vi "MB Update Registers.vi"(8 "error in (no error)":errorcluster, 11 "Modbus Data Unit In":T1={"Function Code"=1, "Data"=[]} {"Function Code" items=["Read Coils"=1, "Read Discrete Inputs"=2, "Read Holding Registers"=3, "Read Input Registers"=4, "Write Single Coil"=5, "Write Single Register"=6, "Read Exception Status"=7, "Write Multiple Coils"=15, "Write Multiple Registers"=16]; "Data" format="%.0x"}) -> (0 "error out":errorcluster, 3 "Modbus Data Unit Out":T1={"Function Code"=1, "Data"=[]} {"Function Code" items=["Read Coils"=1, "Read Discrete Inputs"=2, "Read Holding Registers"=3, "Read Input Registers"=4, "Write Single Coil"=5, "Write Single Register"=6, "Read Exception Status"=7, "Write Multiple Coils"=15, "Write Multiple Registers"=16]; "Data" format="%.0x"})   [LabVIEW 2023, in "Voegtlin_NI_SMART_Modbus_Drivers.lvlib"]
uses:
  Voegtlin_NI_SMART_Modbus_Drivers.lvlib
  MB Modbus Data Unit.ctl
  MB Globals.vi
panel:
  # "VI Name: MB Serial Master Transceive.vi\nPurpose: Performs a MODBUS query and format\nMODBUS Data Unit for the answer.\nReentrant."
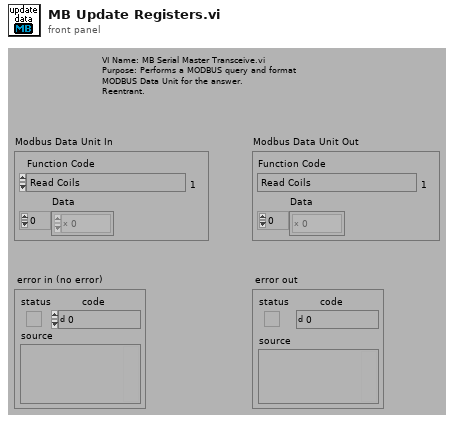
[diagram p1: front panel]
types:
  T1 = typedef "Voegtlin_NI_SMART_Modbus_Drivers.lvlib/MB Modbus Data Unit.ctl" = cluster{"Function Code":u8, "Data":u8[]}
  T2 = enum16{"Discrete Inputs", "Coils", "Input Registers", "Holding Registers"}
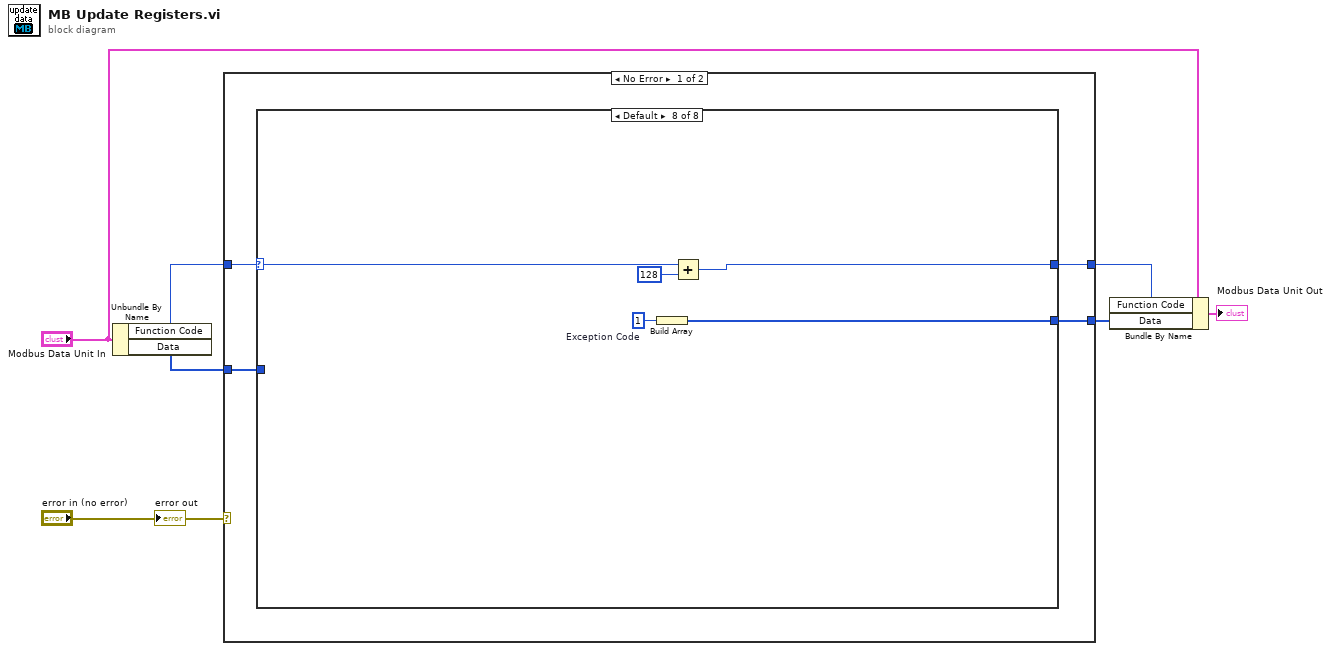
[diagram p0: block diagram]
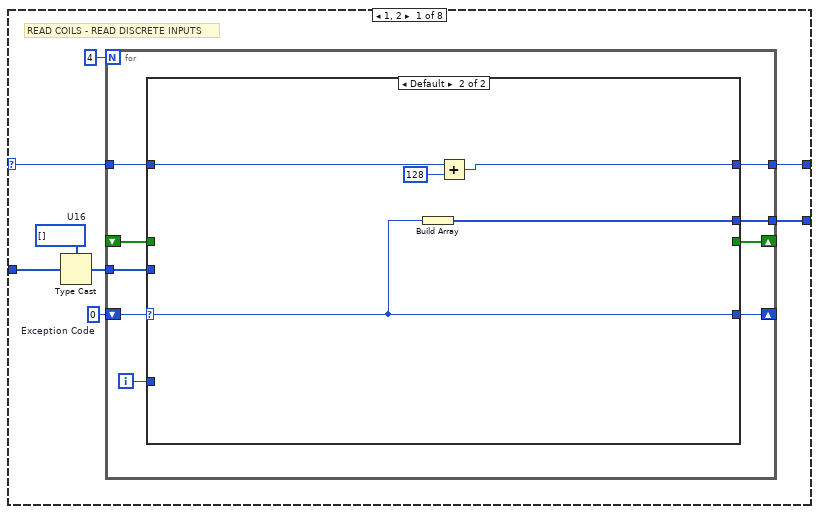
[diagram p2: hidden frame]
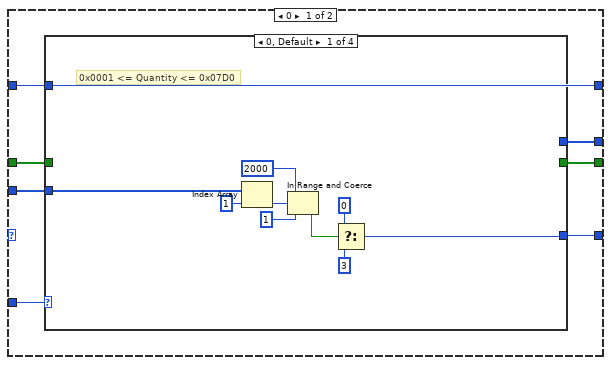
[diagram p3: hidden frame]
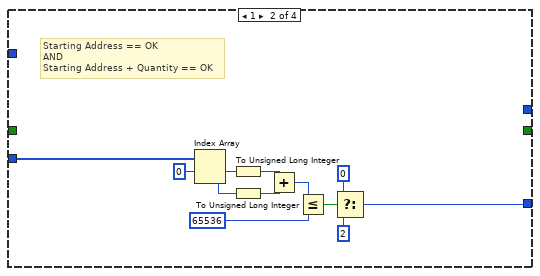
[diagram p4: hidden frame]
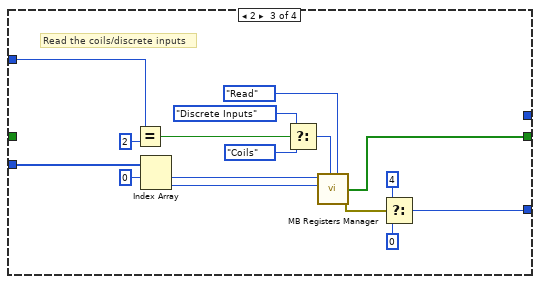
[diagram p5: hidden frame]
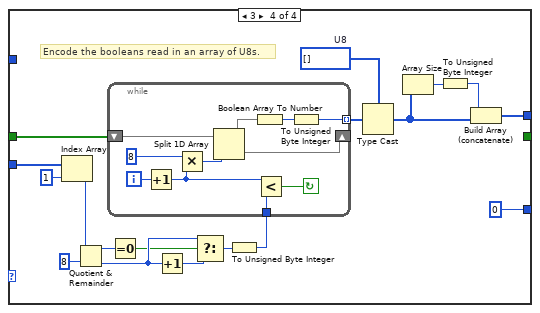
[diagram p6: hidden frame]
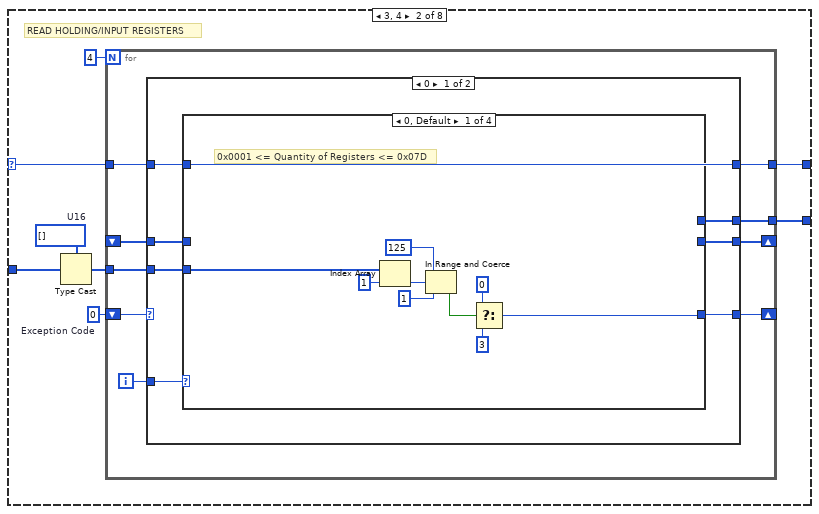
[diagram p7: hidden frame]
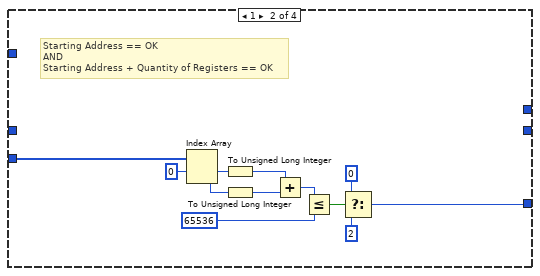
[diagram p8: hidden frame]
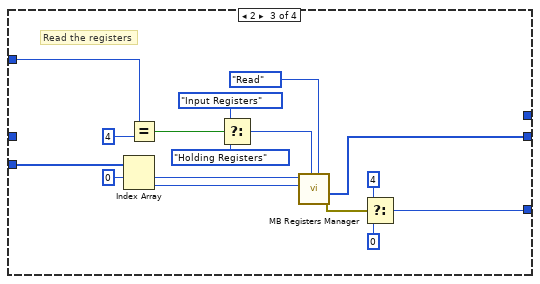
[diagram p9: hidden frame]
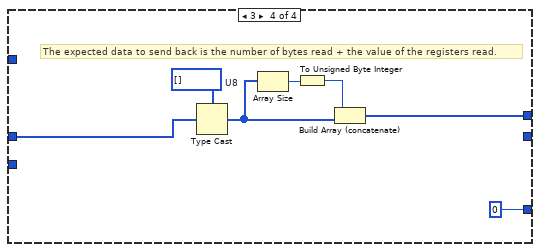
[diagram p10: hidden frame]
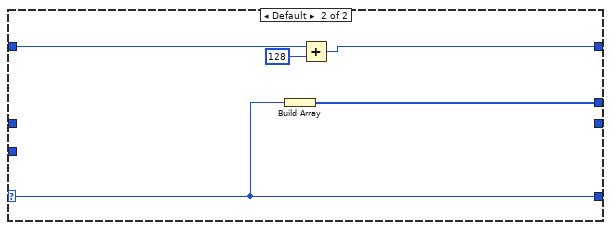
[diagram p11: hidden frame]
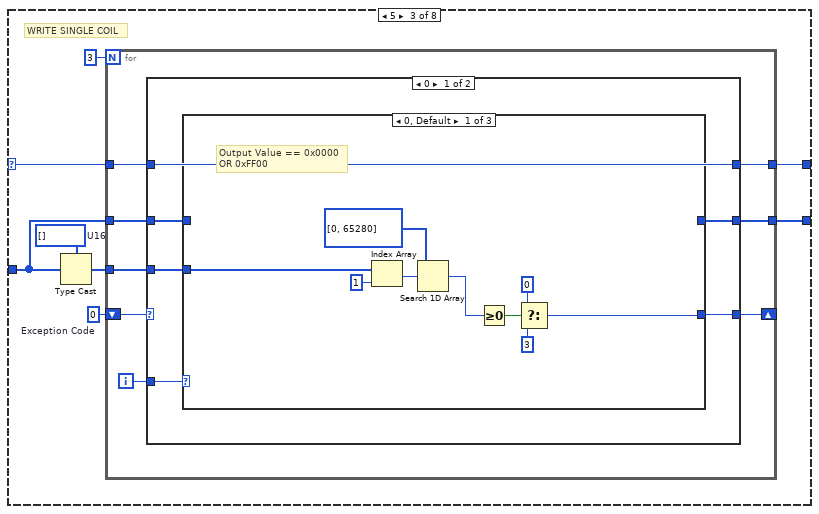
[diagram p12: hidden frame]
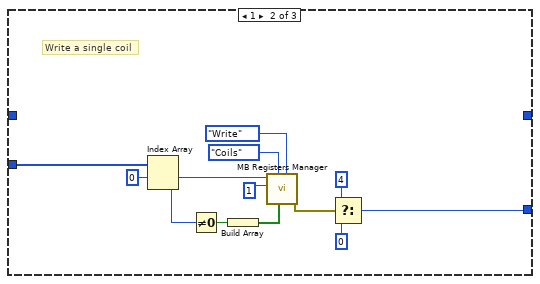
[diagram p13: hidden frame]
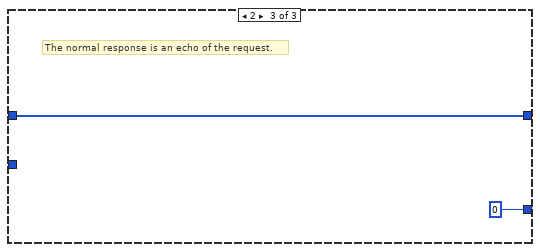
[diagram p14: hidden frame]
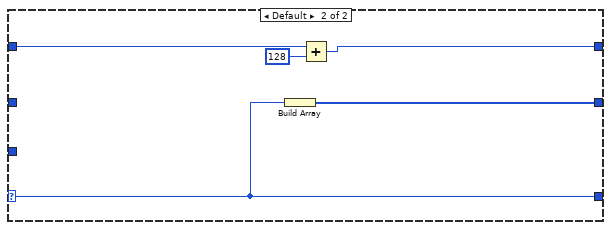
[diagram p15: hidden frame]
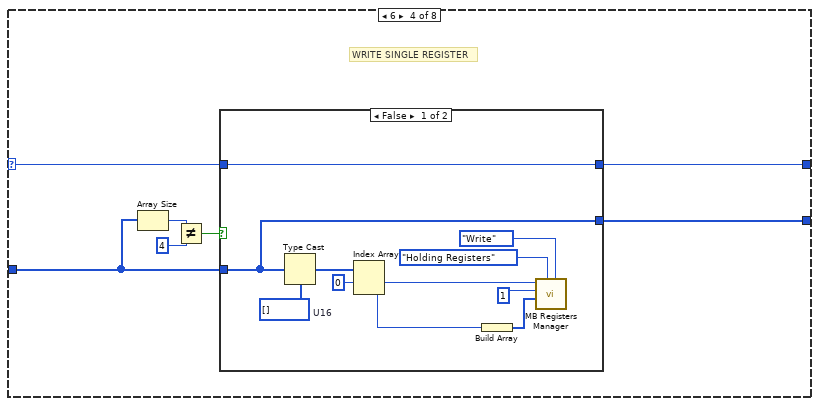
[diagram p16: hidden frame]
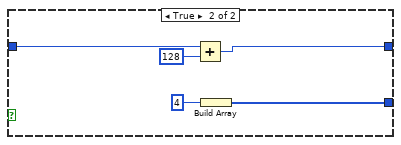
[diagram p17: hidden frame]
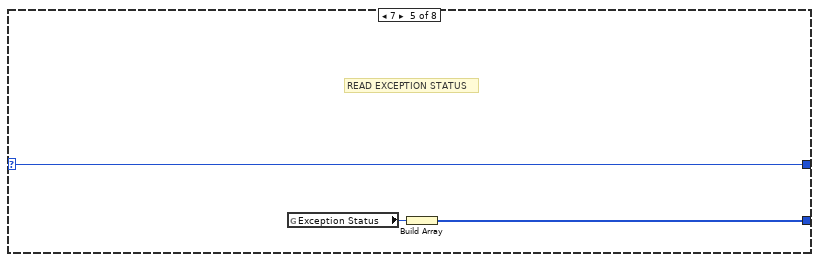
[diagram p18: hidden frame]
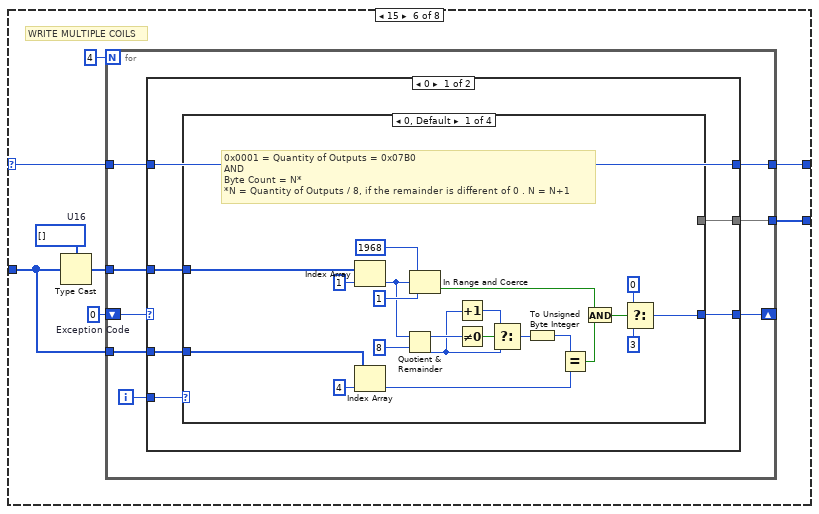
[diagram p19: hidden frame]
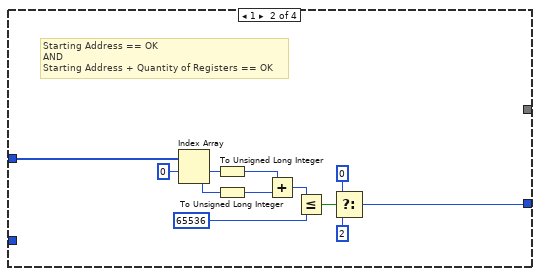
[diagram p20: hidden frame]
diagram:
  n1 = Unbundle By Name("Modbus Data Unit In") -> ("Function Code"=w3:u8, "Data"=w7:u8[])
  n2 = case shown="No Error" "error in (no error)" {
    tunnel: [w11 w421] -> w5
    tunnel: w7 -> [w10 w421]
    tunnel: w3 -> [w9 w420]
    tunnel: [w8 w420] -> w2
    frame No Error {
      n3 = case shown="Default" w9 {
        selector: w9 -> [w12 w107 w181 w237 w255 w258 w342 w418]
        tunnel: w10 -> [w16 w111 w180 w234 _ w257 w341 _]
        tunnel: [w15 w110 w184 w235 w256 w261 w345 w416] -> w11
        tunnel: [w13 w108 w182 w236 w255 w259 w343 w417] -> w8
        frame 1, 2 {
          w18 = u16[] []  # U16
          w19 = u8 0  # Exception Code
          # "READ COILS - READ DISCRETE INPUTS"
          n4 = Type Cast(type=w18, x=w16) -> (*(type *) &x=w17:u16[])
          n5 = for {
            N: 4 -> [_]
            shift-right: [w26] -> _
            shift-left: w19 -> [w28]
            tunnel: w17 -> [w27]
            shift-right: [w25] -> _
            shift-left: _ -> [w24]
            tunnel: [w23] -> w15
            tunnel: [w21] -> w13
            tunnel: w12 -> [w20]
            i -> [w22]
            n6 = case shown="Default" w28 {
              selector: w28 -> [_ w106]
              tunnel: w27 -> [w35 _]
              tunnel: [w34 w106] -> w26
              tunnel: [w33 _] -> w25
              tunnel: w24 -> [w32 _]
              tunnel: [w31 w105] -> w23
              tunnel: w22 -> [w30 _]
              tunnel: [w29 w102] -> w21
              tunnel: w20 -> [w29 w104]
              frame 0 {
                n7 = case shown="0, Default" w30 {
                  tunnel: w35 -> [w43 w55 w71 w89]
                  tunnel: [w38 w54 w63 u8 0] -> w34
                  tunnel: [_ _ w67 _] -> w33
                  tunnel: w32 -> [_ _ _ w75]
                  tunnel: [_ _ _ w74] -> w31
                  tunnel: w29 -> [_ _ w62 _]
                  frame 0, Default {
                    # "0x0001 <= Quantity <= 0x07D0"
                    n8 = Index Array(array=w43, index=1) -> (element=w42:u16)
                    n9 = In Range and Coerce(upper limit=u16 2000, x=w42, lower limit=u16 1) -> (In Range?=w39:bool)  [unwired: 1 out]
                    n10 = Select(t=u8 0, s=w39, f=u8 3) -> (s? t:f=w38:u8)
                  }
                  frame 1 {
                    # "Starting Address == OK\nAND\nStarting Address + Quantity == OK"
                    n11 = Index Array(array=w55, index #1=0 ("index")) -> (element #1=w51:u16, element #2=w48:u16)  [unwired: 1 in]
                    n12 = To Unsigned Long Integer(number=w51) -> (unsigned 32bit integer=w46:u32)
                    n13 = To Unsigned Long Integer(number=w48) -> (unsigned 32bit integer=w47:u32)
                    n14 = Add(x=w46, y=w47) -> (x+y=w50:u32)
                    n15 = Less Or Equal?(x=w50, y=u32 65536 ("upper limit")) -> (x <= y?=w45:bool)
                    n16 = Select(t=u8 0, s=w45, f=u8 2) -> (s? t:f=w54:u8)
                  }
                  frame 2 {
                    # "Read the coils/discrete inputs"
                    n17 = Equal?(x=w62, y=u8 2) -> (x = y?=w60:bool)
                    n18 = Index Array(array=w71, index #1=0 ("index")) -> (element #1=w69:u16, element #2=w68:u16)  [unwired: 1 in]
                    n19 = Select(t=T2."Discrete Inputs" ("Table"), s=w60, f=T2."Coils" ("Table")) -> (s? t:f=w57:T2)
                    n20 = call "MB Registers Manager.vi"("Function"=enum16{"Init", "Read", "Write", "Read All"}."Read", "Table"=w57, "Length"=w68, "Start Address"=w69) -> ("error out"=w66:errorcluster, "Bits out"=w67:bool[])  [unwired: 3 in, 3 out]
                    n21 = Select(t=u8 4, s=w66, f=u8 0) -> (s? t:f=w63:u8)
                  }
                  frame 3 {
                    w77 = u8[] []  # U8
                    # "Encode the booleans read in an array of U8s."
                    n22 = Index Array(array=w89, index=1) -> (element=w82:u16)
                    n23 = Quotient & Remainder(x=w82, y=u16 8) -> (x-y*floor(x/y)=w84:u16, floor(x/y)=w87:u16)
                    n24 = Equal To 0?(x=w84) -> (x = 0?=w85:bool)
                    n25 = Increment(x=w87) -> (x+1=w86:u16)
                    n26 = Select(t=w87, s=w85, f=w86) -> (s? t:f=w88:u16)
                    n27 = To Unsigned Byte Integer(number=w88) -> (unsigned 8bit integer=w76:u8)
                    n28 = while {
                      shift-left: w75 -> [w92]
                      shift-right: [w93] -> _
                      tunnel: [w100] -> w81 mode=indexing
                      tunnel: w76 -> [w91]
                      i -> [w97]
                      stop <- w99 continue-if-true
                      n29 = Increment(x=w97) -> (x+1=w96:i32)
                      n30 = Multiply(x=8, y=w96) -> (x*y=w94:i32)
                      n31 = Split 1D Array(array=w92, index=w94) -> (first subarray=w98:bool[], second subarray=w93:bool[])
                      n32 = Boolean Array To Number(Boolean array=w98) -> (number=w101:u32)
                      n33 = Less?(x=w96, y=w91) -> (x < y?=w99:bool)
                      n34 = To Unsigned Byte Integer(number=w101) -> (unsigned 8bit integer=w100:u8)
                    }
                    n35 = Type Cast(type=w77, x=w81) -> (*(type *) &x=w79:u8[])
                    n36 = Array Size(array=w79) -> (size(s)=w80:i32)
                    n37 = To Unsigned Byte Integer(number=w80) -> (unsigned 8bit integer=w78:u8)
                    n38 = Build Array (concatenate)(w78, w79) -> (w74:u8[])
                  }
                }
              }
              frame Default {
                n39 = Build Array(w106) -> (w105:u8[])
                n40 = Add(x=w104, y=u8 128) -> (x+y=w102:u8)
              }
            }
          }
        }
        frame 3, 4 {
          w113 = u16[] []  # U16
          w114 = u8 0  # Exception Code
          # "READ HOLDING/INPUT REGISTERS"
          n41 = Type Cast(type=w113, x=w111) -> (*(type *) &x=w112:u16[])
          n42 = for {
            N: 4 -> [_]
            shift-right: [w121] -> _
            shift-left: w114 -> [w123]
            tunnel: w112 -> [w122]
            shift-right: [w120] -> _
            shift-left: _ -> [w119]
            tunnel: [w118] -> w110
            tunnel: [w116] -> w108
            tunnel: w107 -> [w115]
            i -> [w117]
            n43 = case shown="0" w123 {
              selector: w123 -> [_ w179]
              tunnel: w122 -> [w130 _]
              tunnel: [w129 w179] -> w121
              tunnel: [w128 _] -> w120
              tunnel: w119 -> [w127 _]
              tunnel: [w126 w178] -> w118
              tunnel: w117 -> [w125 _]
              tunnel: [w124 w175] -> w116
              tunnel: w115 -> [w124 w177]
              frame 0 {
                n44 = case shown="0, Default" w125 {
                  tunnel: w130 -> [w138 w150 w166 _]
                  tunnel: [w133 w149 w159 u8 0] -> w129
                  tunnel: [_ _ w158 _] -> w128
                  tunnel: w127 -> [_ _ _ w168]
                  tunnel: [_ _ _ w169] -> w126
                  tunnel: w124 -> [_ _ w157 _]
                  frame 0, Default {
                    # "0x0001 <= Quantity of Registers <= 0x07D"
                    n45 = Index Array(array=w138, index=1) -> (element=w137:u16)
                    n46 = In Range and Coerce(upper limit=u16 125, x=w137, lower limit=u16 1) -> (In Range?=w134:bool)  [unwired: 1 out]
                    n47 = Select(t=u8 0, s=w134, f=u8 3) -> (s? t:f=w133:u8)
                  }
                  frame 1 {
                    # "Starting Address == OK\nAND\nStarting Address + Quantity of Registers == OK"
                    n48 = Index Array(array=w150, index #1=0 ("index")) -> (element #1=w146:u16, element #2=w143:u16)  [unwired: 1 in]
                    n49 = To Unsigned Long Integer(number=w146) -> (unsigned 32bit integer=w141:u32)
                    n50 = To Unsigned Long Integer(number=w143) -> (unsigned 32bit integer=w142:u32)
                    n51 = Add(x=w141, y=w142) -> (x+y=w145:u32)
                    n52 = Less Or Equal?(x=w145, y=u32 65536 ("upper limit")) -> (x <= y?=w140:bool)
                    n53 = Select(t=u8 0, s=w140, f=u8 2) -> (s? t:f=w149:u8)
                  }
                  frame 2 {
                    # "Read the registers"
                    n54 = Index Array(array=w166, index #1=0 ("index")) -> (element #1=w164:u16, element #2=w163:u16)  [unwired: 1 in]
                    n55 = Equal?(x=w157, y=u8 4) -> (x = y?=w155:bool)
                    n56 = Select(t=T2."Input Registers" ("Table"), s=w155, f=T2."Holding Registers" ("Table")) -> (s? t:f=w152:T2)
                    n57 = call "MB Registers Manager.vi"("Function"=enum16{"Init", "Read", "Write", "Read All"}."Read", "Table"=w152, "Length"=w163, "Start Address"=w164) -> ("error out"=w162:errorcluster, "Words out"=w158:u16[])  [unwired: 3 in, 3 out]
                    n58 = Select(t=u8 4, s=w162, f=u8 0) -> (s? t:f=w159:u8)
                  }
                  frame 3 {
                    w173 = u8[] []  # U8
                    # "The expected data to send back is the number of bytes read + the value of the registers read."
                    n59 = Type Cast(type=w173, x=w168) -> (*(type *) &x=w170:u8[])
                    n60 = Array Size(array=w170) -> (size(s)=w171:i32)
                    n61 = To Unsigned Byte Integer(number=w171) -> (unsigned 8bit integer=w172:u8)
                    n62 = Build Array (concatenate)(w172, w170) -> (w169:u8[])
                  }
                }
              }
              frame Default {
                n63 = Build Array(w179) -> (w178:u8[])
                n64 = Add(x=w177, y=u8 128) -> (x+y=w175:u8)
              }
            }
          }
        }
        frame 5 {
          w186 = u16[] []  # U16
          w187 = u8 0  # Exception Code
          # "WRITE SINGLE COIL"
          n65 = Type Cast(type=w186, x=w180) -> (*(type *) &x=w185:u16[])
          n66 = for {
            N: 3 -> [_]
            shift-right: [w193] -> _
            shift-left: w187 -> [w195]
            tunnel: w185 -> [w194]
            tunnel: [w192] -> w184
            tunnel: [w190] -> w182
            tunnel: w181 -> [w189]
            tunnel: w180 -> [w188]
            i -> [w191]
            n67 = case shown="0" w195 {
              selector: w195 -> [_ w230]
              tunnel: w194 -> [w201 _]
              tunnel: [w200 w230] -> w193
              tunnel: [w199 w229] -> w192
              tunnel: w191 -> [w198 _]
              tunnel: [w197 w226] -> w190
              tunnel: w189 -> [w197 w228]
              tunnel: w188 -> [w196 _]
              frame 0 {
                n68 = case shown="0, Default" w198 {
                  tunnel: w201 -> [w209 w222 _]
                  tunnel: [w208 w215 u8 0] -> w200
                  tunnel: [_ _ w224] -> w199
                  tunnel: w196 -> [_ _ w224]
                  frame 0, Default {
                    # "Output Value == 0x0000\nOR 0xFF00"
                    n69 = Index Array(array=w209, index=1) -> (element=w205:u16)
                    n70 = Search 1D Array(1D array=u16[] [0, 65280], element=w205) -> (index of element=w203:i32)  [unwired: 1 out]
                    n71 = Greater Or Equal To 0?(x=w203) -> (x >= 0?=w202:bool)
                    n72 = Select(t=u8 0, s=w202, f=u8 3) -> (s? t:f=w208:u8)
                  }
                  frame 1 {
                    # "Write a single coil"
                    n73 = Index Array(array=w222, index #1=0 ("index")) -> (element #1=w219:u16, element #2=w213:u16)  [unwired: 1 in]
                    n74 = Not Equal To 0?(x=w213) -> (x != 0?=w214:bool)
                    n75 = Build Array(w214) -> (w212:bool[])
                    n76 = call "MB Registers Manager.vi"("Function"=enum16{"Init", "Read", "Write", "Read All"}."Write", "Bits In"=w212, "Table"=T2."Coils", "Length"=u16 1, "Start Address"=w219) -> ("error out"=w218:errorcluster)  [unwired: 2 in, 4 out]
                    n77 = Select(t=u8 4, s=w218, f=u8 0) -> (s? t:f=w215:u8)
                  }
                  frame 2 {
                    # "The normal response is an echo of the request."
                  }
                }
              }
              frame Default {
                n78 = Build Array(w230) -> (w229:u8[])
                n79 = Add(x=w228, y=u8 128) -> (x+y=w226:u8)
              }
            }
          }
        }
        frame 6 {
          # "WRITE SINGLE REGISTER"
          n80 = Array Size(array=w234) -> (size(s)=w233:i32)
          n81 = Not Equal?(x=w233, y=4) -> (x != y?=w231:bool)
          n82 = case shown="False" w231 {
            tunnel: w234 -> [w238 _]
            tunnel: w237 -> [w239 w252]
            tunnel: [w239 w251] -> w236
            tunnel: [w238 w250] -> w235
            frame False {
              w248 = u16[] []  # U16
              n83 = Type Cast(type=w248, x=w238) -> (*(type *) &x=w247:u16[])
              n84 = Index Array(array=w247, index #1=0 ("index")) -> (element #1=w243:u16, element #2=w241:u16)  [unwired: 1 in]
              n85 = Build Array(w241) -> (w240:u16[])
              n86 = call "MB Registers Manager.vi"("Function"=enum16{"Init", "Read", "Write", "Read All"}."Write", "Table"=T2."Holding Registers", "Words In"=w240, "Length"=u16 1, "Start Address"=w243) -> ()  [unwired: 2 in, 5 out]
            }
            frame True {
              n87 = Add(x=w252, y=u8 128) -> (x+y=w251:u8)
              n88 = Build Array(u8 4 ("element")) -> (w250:u8[])
            }
          }
        }
        frame 7 {
          # "READ EXCEPTION STATUS"
          n89 = global read "MB Globals.vi" "Exception Status"() -> (w254:u8)
          n90 = Build Array(w254) -> (w256:u8[])
        }
        frame 15 {
          w263 = u16[] []  # U16
          w264 = u8 0  # Exception Code
          # "WRITE MULTIPLE COILS"
          n91 = Type Cast(type=w263, x=w257) -> (*(type *) &x=w262:u16[])
          n92 = for {
            N: 4 -> [_]
            shift-right: [w270] -> _
            shift-left: w264 -> [w272]
            tunnel: w262 -> [w271]
            tunnel: [w269] -> w261
            tunnel: [w267] -> w259
            tunnel: w258 -> [w266]
            tunnel: w257 -> [w265]
            i -> [w268]
            n93 = case shown="0" w272 {
              selector: w272 -> [_ w340]
              tunnel: w271 -> [w278 _]
              tunnel: [w277 w340] -> w270
              tunnel: [w276 w339] -> w269
              tunnel: w268 -> [w275 _]
              tunnel: [w274 w336] -> w267
              tunnel: w266 -> [w274 w338]
              tunnel: w265 -> [w273 _]
              frame 0 {
                n94 = case shown="0, Default" w275 {
                  tunnel: w278 -> [w293 w310 w326 _]
                  tunnel: [w296 w309 w319 u8 0] -> w277
                  tunnel: [_ _ _ w332] -> w276
                  tunnel: w273 -> [w283 _ w313 w333]
                  frame 0, Default {
                    # "0x0001 = Quantity of Outputs = 0x07B0\nAND\nByte Count = N*\n*N = Quantity of Outputs / 8, if the remainder is different of 0 . N = N+1"
                    n95 = Index Array(array=w293, index=1) -> (element=w291:u16)
                    n96 = Index Array(array=w283, index=4) -> (element=w287:u8)
                    n97 = Quotient & Remainder(x=w291, y=u16 8) -> (x-y*floor(x/y)=w280:u16, floor(x/y)=w279:u16)
                    n98 = In Range and Coerce(upper limit=u16 1968, x=w291, lower limit=u16 1) -> (In Range?=w285:bool)  [unwired: 1 out]
                    n99 = Increment(x=w279) -> (x+1=w288:u16)
                    n100 = Not Equal To 0?(x=w280) -> (x != 0?=w289:bool)
                    n101 = Select(t=w288, s=w289, f=w279) -> (s? t:f=w281:u16)
                    n102 = To Unsigned Byte Integer(number=w281) -> (unsigned 8bit integer=w282:u8)
                    n103 = Equal?(x=w282, y=w287) -> (x = y?=w286:bool)
                    n104 = And(x=w285, y=w286) -> (x .and. y?=w284:bool)
                    n105 = Select(t=u8 0, s=w284, f=u8 3) -> (s? t:f=w296:u8)
                  }
                  frame 1 {
                    # "Starting Address == OK\nAND\nStarting Address + Quantity of Registers == OK"
                    n106 = Index Array(array=w310, index #1=0 ("index")) -> (element #1=w306:u16, element #2=w303:u16)  [unwired: 1 in]
                    n107 = To Unsigned Long Integer(number=w306) -> (unsigned 32bit integer=w301:u32)
                    n108 = To Unsigned Long Integer(number=w303) -> (unsigned 32bit integer=w302:u32)
                    n109 = Add(x=w301, y=w302) -> (x+y=w305:u32)
                    n110 = Less Or Equal?(x=w305, y=u32 65536 ("upper limit")) -> (x <= y?=w300:bool)
                    n111 = Select(t=u8 0, s=w300, f=u8 2) -> (s? t:f=w309:u8)
                  }
                  frame 2 {
                    # "Write multiple coils"
                    n112 = Array Subset(array=w313, index=5) -> (w316:u8[])  [unwired: 1 in]
                    n113 = Index Array(array=w326, index #1=0 ("index")) -> (element #1=w323:u16, element #2=w314:u16)  [unwired: 1 in]
                    n114 = for {
                      tunnel: w316 -> [w331] mode=indexing
                      shift-right: [w328] -> w318
                      shift-left: bool[] [] ("words out") -> [w329]
                      n115 = Number To Boolean Array(number=w331) -> (Boolean array=w330:bool[])
                      n116 = Build Array (concatenate)(w329, w330) -> (w328:bool[])
                    }
                    n117 = Array Subset(array=w318, length=w314) -> (w312:bool[])  [unwired: 1 in]
                    n118 = call "MB Registers Manager.vi"("Function"=enum16{"Init", "Read", "Write", "Read All"}."Write", "Bits In"=w312, "Table"=T2."Coils", "Length"=w314, "Start Address"=w323) -> ("error out"=w322:errorcluster)  [unwired: 2 in, 4 out]
                    n119 = Select(t=u8 4, s=w322, f=u8 0) -> (s? t:f=w319:u8)
                  }
                  frame 3 {
                    # "The normal response returns the function code, starting address, and quantity of coils forced."
                    n120 = Array Subset(array=w333, length=4) -> (w332:u8[])  [unwired: 1 in]
                  }
                }
              }
              frame Default {
                n121 = Build Array(w340) -> (w339:u8[])
                n122 = Add(x=w338, y=u8 128) -> (x+y=w336:u8)
              }
            }
          }
        }
        frame 16 {
          w347 = u16[] []  # U16
          w348 = u8 0  # Exception Code
          # "WRITE MULTIPLE REGISTERS"
          n123 = Type Cast(type=w347, x=w341) -> (*(type *) &x=w346:u16[])
          n124 = for {
            N: 4 -> [_]
            shift-right: [w354] -> _
            shift-left: w348 -> [w356]
            tunnel: w346 -> [w355]
            tunnel: [w353] -> w345
            tunnel: [w351] -> w343
            tunnel: w342 -> [w350]
            tunnel: w341 -> [w349]
            i -> [w352]
            n125 = case shown="Default" w356 {
              selector: w356 -> [_ w414]
              tunnel: w355 -> [w362 _]
              tunnel: [w361 w414] -> w354
              tunnel: [w360 w413] -> w353
              tunnel: w352 -> [w359 _]
              tunnel: [w358 w410] -> w351
              tunnel: w350 -> [w358 w412]
              tunnel: w349 -> [w357 _]
              frame 0 {
                n126 = case shown="0, Default" w359 {
                  tunnel: w362 -> [w372 w389 w404 _]
                  tunnel: [w375 w388 w397 u8 0] -> w361
                  tunnel: [_ _ _ w406] -> w360
                  tunnel: w357 -> [w366 _ w394 w407]
                  frame 0, Default {
                    # "0x0001 = Quantity of Outputs = 0x0078\nAND\nByte Count = Byte Count == Quantity of Registers x 2"
                    n127 = Index Array(array=w372, index=1) -> (element=w365:u16)
                    n128 = Index Array(array=w366, index=4) -> (element=w370:u8)
                    n129 = To Unsigned Word Integer(number=w370) -> (unsigned 16bit integer=w363:u16)
                    n130 = In Range and Coerce(upper limit=u16 120, x=w365, lower limit=u16 1) -> (In Range?=w368:bool)  [unwired: 1 out]
                    n131 = expression code="x*2"(w365) -> (w364:u16)
                    n132 = Equal?(x=w364, y=w363) -> (x = y?=w369:bool)
                    n133 = And(x=w368, y=w369) -> (x .and. y?=w367:bool)
                    n134 = Select(t=u8 0, s=w367, f=u8 3) -> (s? t:f=w375:u8)
                  }
                  frame 1 {
                    # "Starting Address == OK\nAND\nStarting Address + Quantity of Registers == OK"
                    n135 = Index Array(array=w389, index #1=0 ("index")) -> (element #1=w385:u16, element #2=w382:u16)  [unwired: 1 in]
                    n136 = To Unsigned Long Integer(number=w385) -> (unsigned 32bit integer=w380:u32)
                    n137 = To Unsigned Long Integer(number=w382) -> (unsigned 32bit integer=w381:u32)
                    n138 = Add(x=w380, y=w381) -> (x+y=w384:u32)
                    n139 = Less Or Equal?(x=w384, y=u32 65536 ("upper limit")) -> (x <= y?=w379:bool)
                    n140 = Select(t=u8 0, s=w379, f=u8 2) -> (s? t:f=w388:u8)
                  }
                  frame 2 {
                    w392 = u16[] []  # U16
                    # "Write Multiple registers"
                    n141 = Array Subset(array=w394, index=5) -> (w393:u8[])  [unwired: 1 in]
                    n142 = Index Array(array=w404, index #1=0 ("index")) -> (element #1=w401:u16, element #2=w395:u16)  [unwired: 1 in]
                    n143 = Type Cast(type=w392, x=w393) -> (*(type *) &x=w391:u16[])
                    n144 = call "MB Registers Manager.vi"("Function"=enum16{"Init", "Read", "Write", "Read All"}."Write", "Table"=T2."Holding Registers", "Words In"=w391, "Length"=w395, "Start Address"=w401) -> ("error out"=w400:errorcluster)  [unwired: 2 in, 4 out]
                    n145 = Select(t=u8 4, s=w400, f=u8 0) -> (s? t:f=w397:u8)
                  }
                  frame 3 {
                    # "The normal response returns the function code, starting address, and quantity of registers written."
                    n146 = Array Subset(array=w407, length=4) -> (w406:u8[])  [unwired: 1 in]
                  }
                }
              }
              frame Default {
                n147 = Build Array(w414) -> (w413:u8[])
                n148 = Add(x=w412, y=u8 128) -> (x+y=w410:u8)
              }
            }
          }
        }
        frame Default {
          w415 = u8 1  # Exception Code
          n149 = Build Array(w415) -> (w416:u8[])
          n150 = Add(x=w418, y=u8 128) -> (x+y=w417:u8)
        }
      }
    }
    frame Error {
    }
  }
  n151 = Bundle By Name(cluster="Modbus Data Unit In", "Function Code"=w2, "Data"=w5) -> (→"Modbus Data Unit Out":T1)
  "error out" <- "error in (no error)"
